vi "Close Client.vi"(8 "error in":errorcluster, 11 "ClientID in":T1) -> (0 "error out":errorcluster)   [LabVIEW 2019, in "gprc-lvsupport.lvlib"]
uses:
  gprc-lvsupport.lvlib
  Shared/grpcId.ctl
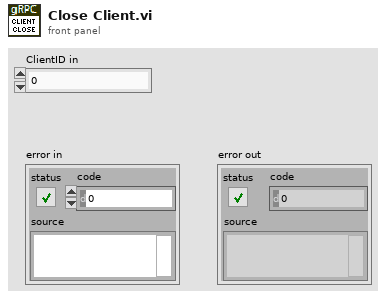
[diagram p1: front panel]
types:
  T1 = typedef "gprc-lvsupport.lvlib/grpcId.ctl" = u64
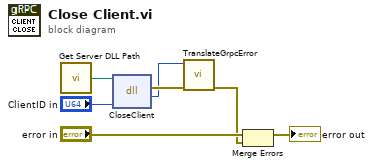
[diagram p0: block diagram]
diagram:
  n1 = call "Get Server DLL Path.vi"() -> ("Server dll path"=w6:path)
  n2 = dll-call lib="?" fn="CloseClient"(path in=w6, "clientId"="ClientID in") -> (error out=w7:errorcluster, "return type"=w4:i32)  [unwired: 3 in, 1 out]
  n3 = call "TranslateGrpcError.vi"("error in"=w7, "Error Code"=w4) -> ("error out"=w2:errorcluster)  [unwired: 9 in]
  n4 = Merge Errors("error in", w2) -> (→"error out":errorcluster)
